vi "CloseConnection.vi"(8 "error in (no error)":errorcluster, 10 "timeout [ms]":i32=5000, 11 "Communicator in":refnum<class "Communicator.lvclass">) -> (0 "error out":errorcluster, 3 "Communicator out":refnum<class "Communicator.lvclass">)   [LabVIEW 2023, in "Communicator.lvclass"]
doc: "Closes the websocket connection."
uses:
  Communicator.lvclass
  Communicator.lvclass/Communicator.ctl
  <vilib>/MediaMongrels Ltd/WebSockets/WebSockets/WebSocket Client/WebSocket Client.lvclass
panel:
  # "Connector Pane"
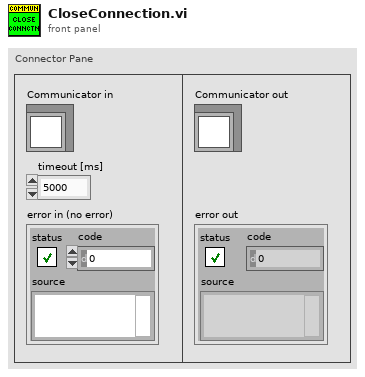
[diagram p1: front panel]
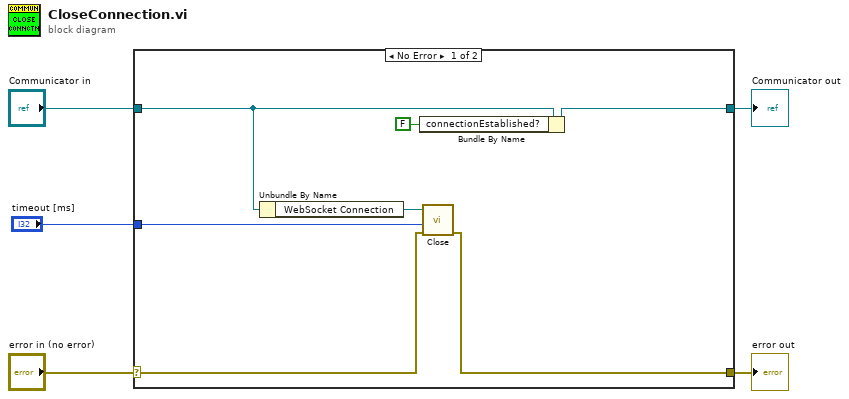
[diagram p0: block diagram]
diagram:
  n1 = case shown="No Error" "error in (no error)" {
    selector: "error in (no error)" -> [w12 w14]
    tunnel: [w11 w14] -> w4
    tunnel: [w7 w13] -> w2
    tunnel: "Communicator in" -> [w10 w13]
    tunnel: "timeout [ms]" -> [w8 _]
    frame No Error {
      n2 = Unbundle By Name(w10) -> ("WebSocket Connection"=w9:refnum<class "WebSocket Client.lvclass">)
      n3 = Bundle By Name(cluster=w10, "connectionEstablished?"=FALSE) -> (w7:refnum<class "Communicator.lvclass">)
      n4 = call-dynamic "Close.vi"("error in (no error)"=w12, "timeout ms (5000)"=w8, "WebSocket in"=w9) -> ("error out"=w11:errorcluster)  [unwired: 8 in]
    }
    frame Error {
    }
  }
  "error out" <- w4
  "Communicator out" <- w2
